vi "GetOrCalculateTime VolumeOrTime.vi"(1 "Units":string, 2 "Target Volume":dbl, 3 "Target Time":dbl, 4 "Flow Rate":dbl, 5 "State?":bool) -> (0 "Time Output":dbl)   [LabVIEW 2020]
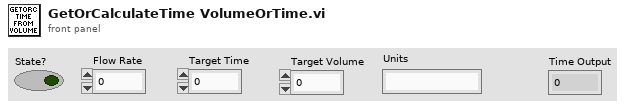
[diagram p1: front panel]
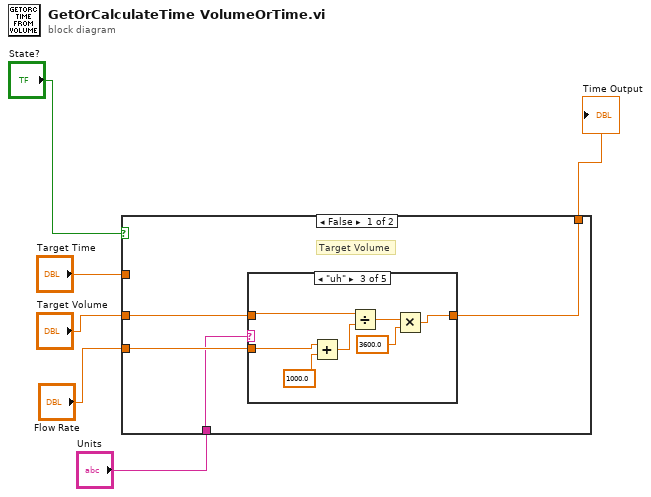
[diagram p0: block diagram]
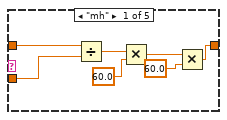
[diagram p2: hidden frame]
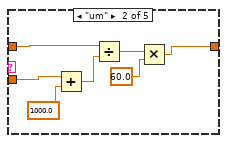
[diagram p3: hidden frame]
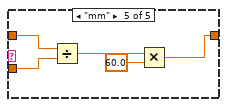
[diagram p5: hidden frame]
diagram:
  n1 = case shown="False" "State?" {
    tunnel: [w7 w38] -> w5
    tunnel: "Target Time" -> [_ w38]
    tunnel: "Target Volume" -> [w10 _]
    tunnel: "Flow Rate" -> [w9 _]
    tunnel: "Units" -> [w8 _]
    frame False {
      # "Target Volume"
      n2 = case shown="\"uh\"" w8 {
        tunnel: w10 -> [w13 w22 w27 w32 w37]
        tunnel: [w16 w21 w25 w32 w34] -> w7
        tunnel: w9 -> [w12 w20 w26 _ w36]
        frame "mh" {
          n3 = Divide(x=w13, y=w12) -> (x/y=w14:dbl)
          n4 = Multiply(x=w14, y=60.0) -> (x*y=w15:dbl)
          n5 = Multiply(x=w15, y=60.0) -> (x*y=w16:dbl)
        }
        frame "um" {
          n6 = Add(x=w20, y=1000.0) -> (x+y=w18:dbl)
          n7 = Divide(x=w22, y=w18) -> (x/y=w24:dbl)
          n8 = Multiply(x=w24, y=60.0) -> (x*y=w21:dbl)
        }
        frame "uh" {
          n9 = Add(x=w26, y=1000.0) -> (x+y=w28:dbl)
          n10 = Divide(x=w27, y=w28) -> (x/y=w31:dbl)
          n11 = Multiply(x=w31, y=3600.0) -> (x*y=w25:dbl)
        }
        frame Default {
        }
        frame "mm" {
          n12 = Divide(x=w37, y=w36) -> (x/y=w35:dbl)
          n13 = Multiply(x=w35, y=60.0) -> (x*y=w34:dbl)
        }
      }
    }
    frame True {
      # "Target Time"
    }
  }
  "Time Output" <- w5
